vi "DIYTrigger (subVI).vi"(6 "Pre Samples":i32, 7 "Ä²µo¶b":enum32{"Channel 1", "Channel 2", "Channel 3"}(ring), 8 "error in (no error)":errorcluster, 9 "Samples to Read":i32, 10 "Trigger Slope":enum16{"Falling Edge", "Rising Edge"}(ring), 11 "Trigger Level":dbl) -> (0 "error out":errorcluster, 1 "trigger detected?":bool, 2 "Section":dynamicdata(waveform), 3 "Enable":bool)   [LabVIEW 2018]
uses:
  <vilib>/measure/mamon.llb/Trigger Detection for 1 Channel.vi
  <vilib>/measure/NI_MAPro.lvlib
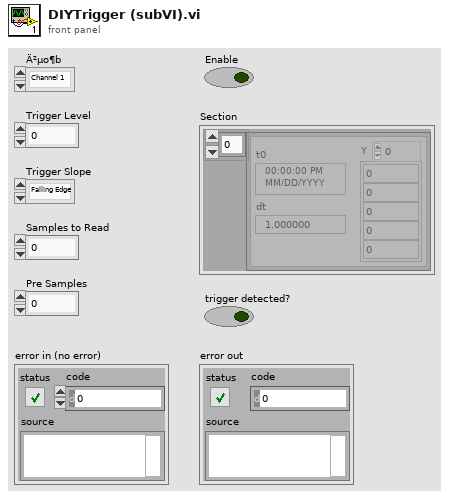
[diagram p1: front panel]
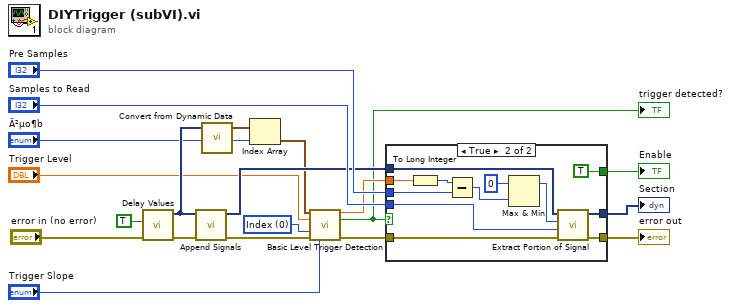
[diagram p0: block diagram]
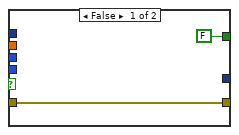
[diagram p2: hidden frame]
diagram:
  w5 = u16 0 items=["Index", "Time"] ("location mode")
  n1 = call "Delay Values"("error in (no error)"="error in (no error)", "Enable"=TRUE) -> ("error out"=w12:errorcluster, "Delayed Signals"=w11:dynamicdata)  [unwired: 8 in]
  n2 = call "Append Signals"("error in (no error)"=w12, "Input Signal A"=w11) -> ("error out"=w13:errorcluster, "Appended Signals"=w15:dynamicdata)  [unwired: 8 in]
  n3 = call "Convert from Dynamic Data"("Dynamic Data Type"=w11) -> ("Array of Waveform"=w1:waveform(dbl)[])  [unwired: 3 in]
  n4 = Index Array(array=w1, index="Ä²µo¶b") -> (element=w2:waveform(dbl))
  n5 = call-poly <vilib>:"Basic Level Trigger Detection.vi"("signal in"=w2, "level"="Trigger Level", "location mode"=w5, "error in (no error)"=w13, "trigger slope"="Trigger Slope") -> ("trigger location"=w8:dbl, "trigger detected?"=w7:bool, "error out"=w14:errorcluster)  [unwired: 8 in]
  "trigger detected?" <- w7
  n6 = case shown="True" w7 {
    tunnel: w8 -> [_ w33]
    tunnel: w14 -> [w21 w34]
    tunnel: w15 -> [_ w28]
    tunnel: [FALSE ("Enable") TRUE ("Enable")] -> w16
    tunnel: [w21 w31] -> w17
    tunnel: [_ w29] -> w18
    tunnel: "Pre Samples" -> [_ w26]
    tunnel: "Samples to Read" -> [_ w23]
    frame False {
    }
    frame True {
      n7 = To Long Integer(number=w33) -> (32bit integer=w32:i32)
      n8 = Subtract(x=w32, y=w26) -> (x-y=w27:i32)
      n9 = Max & Min(x=0, y=w27) -> (max(x,y)=w24:i32)  [unwired: 1 out]
      n10 = call "Extract Portion of Signal"("error in (no error)"=w34, "Samples"=w23, "Begin Sample"=w24, "Signals"=w28) -> ("error out"=w31:errorcluster, "Section"=w29:dynamicdata)  [unwired: 6 in]
    }
  }
  "Section" <- w18
  "error out" <- w17
  "Enable" <- w16
